vi "Compute Motor Command From Xbox Data.vi"(1 "Parameters":T3={"Turn deadzone"=10240, "Turn scaling factor"=2000, "Speed scaling factor "=400, "Speed deadzone "=10240}, 2 "Xbox Controller Axis Info":T2={"X axis"=-5590, "Y axis"=-2806, "Z axis"=0, "X axis rotation"=-2901, "Y axis rotation"=-1955, "Z axis rotation"=0, "U axis"=0, "V axis"=0}) -> (0 "Motor Command":T1)   [LabVIEW 2009]
uses:
  Motor Command.ctl
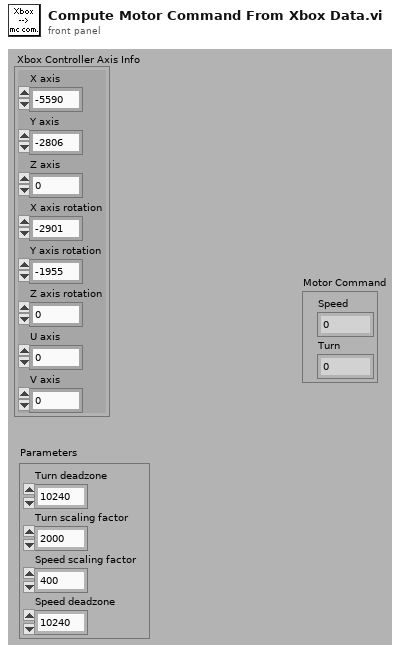
[diagram p1: front panel]
types:
  T1 = typedef "Motor Command.ctl" = cluster{"Speed":i16, "Turn":i16}
  T2 = cluster{"X axis":i32, "Y axis":i32, "Z axis":i32, "X axis rotation":i32, "Y axis rotation":i32, "Z axis rotation":i32, "U axis":i32, "V axis":i32}
  T3 = cluster{"Turn deadzone":i32, "Turn scaling factor":i32, "Speed scaling factor ":i32, "Speed deadzone ":i32}
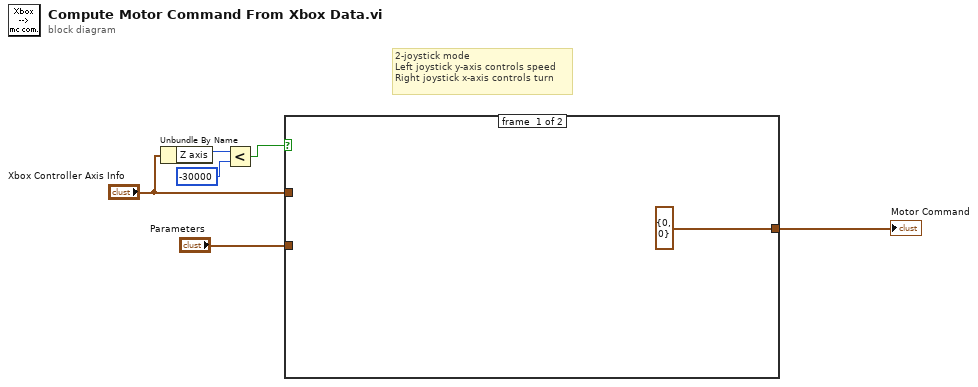
[diagram p0: block diagram]
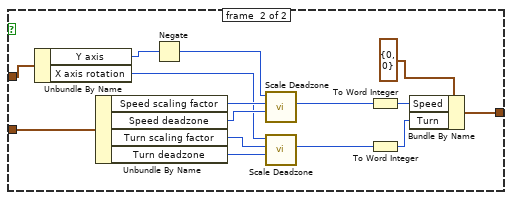
[diagram p2: hidden frame]
diagram:
  # "2-joystick mode\nLeft joystick y-axis controls speed\nRight joystick x-axis controls turn"
  n1 = Unbundle By Name("Xbox Controller Axis Info") -> ("Z axis"=w3:i32)
  n2 = Less?(x=w3, y=-30000) -> (x < y?=w1:bool)
  n3 = case shown="False" w1 {
    tunnel: [T1 {"Speed"=0, "Turn"=0} ("Motor Command") w12] -> w6
    tunnel: "Xbox Controller Axis Info" -> [_ w11]
    tunnel: "Parameters" -> [_ w10]
    frame #0 {
    }
    frame #1 {
      n4 = Unbundle By Name(w11) -> ("Y axis"=w9:i32, "X axis rotation"=w8:i32)
      n5 = Unbundle By Name(w10) -> ("Speed scaling factor"=w18:i32, "Speed deadzone"=w19:i32, "Turn scaling factor"=w20:i32, "Turn deadzone"=w21:i32)
      n6 = Negate(x=w9) -> (-x=w13:i32)
      n7 = call "Scale Deadzone.vi"("deadzone"=w19, "scaling factor"=w18, "input value"=w13) -> ("output value"=w22:i32)  [unwired: 8 in]
      n8 = call "Scale Deadzone.vi"("deadzone"=w21, "scaling factor"=w20, "input value"=w8) -> ("output value"=w17:i32)  [unwired: 8 in]
      n9 = To Word Integer(number=w22) -> (16bit integer=w16:i16)
      n10 = To Word Integer(number=w17) -> (16bit integer=w15:i16)
      n11 = Bundle By Name(cluster=T1 {"Speed"=0, "Turn"=0} ("Motor Command"), "Speed"=w16, "Turn"=w15) -> (w12:T1)
    }
  }
  "Motor Command" <- w6
